vi "Process Motor Status.vi"(8 "error in (no error)":errorcluster, 11 "Motor Error Status":T1) -> (0 "error out":errorcluster, 3 "Error description":string)   [LabVIEW 2012, in "Roboteq.lvlib"]
doc: "Processes the motor status error and outputs a string describing the errors if any."
uses:
  Roboteq.lvlib
  <instrlib>/Dynamixel Motor/Public/Motor Operation/Low Level/Alarm Setting.ctl
  <instrlib>/Dynamixel Motor/Dynamixel Motor.lvlib
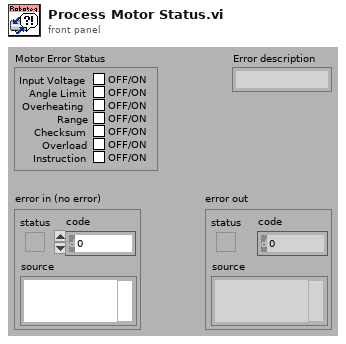
[diagram p1: front panel]
types:
  T1 = typedef "Dynamixel Motor.lvlib/Alarm Setting.ctl" = cluster{"Input Voltage":bool, "Angle Limit":bool, "Overheating ":bool, "Range":bool, "Checksum":bool, "Overload":bool, "Instruction":bool}
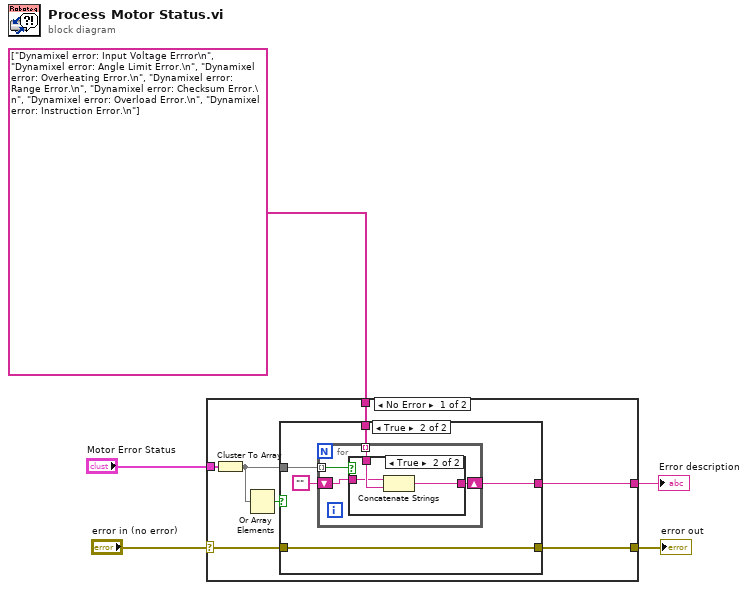
[diagram p0: block diagram]
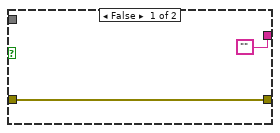
[diagram p2: hidden frame]
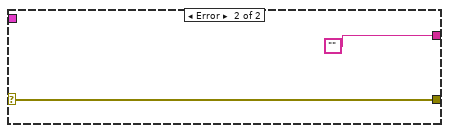
[diagram p4: hidden frame]
diagram:
  n1 = case shown="No Error" "error in (no error)" {
    selector: "error in (no error)" -> [w10 w29]
    tunnel: [w9 w29] -> w4
    tunnel: "Motor Error Status" -> [w12 _]
    tunnel: string[] ["Dynamixel error: Input Voltage Errror\n", "Dynamixel error: Angle Limit Error.\n", "Dynamixel error: Overheating Error.\n", "Dynamixel error: Range Error.\n", "Dynamixel error: Checksum Error.\n", "Dynamixel error: Overload Error.\n", "Dynamixel error: Instruction Error.\n"] -> [w11 _]
    tunnel: [w6 ""] -> w1
    frame No Error {
      n2 = Cluster To Array(cluster=w12) -> (array=w7:bool[])
      n3 = Or Array Elements(Boolean array=w7) -> (logical OR=w8:bool)
      n4 = case shown="True" w8 {
        tunnel: w11 -> [_ w19]
        tunnel: w10 -> [w14 w16]
        tunnel: [w14 w16] -> w9
        tunnel: w7 -> [_ w18]
        tunnel: ["" w15] -> w6
        frame False {
        }
        frame True {
          n5 = for {
            tunnel: w19 -> [w23] mode=indexing
            tunnel: w18 -> [w20] mode=indexing
            shift-right: [w21] -> w15
            shift-left: "" -> [w22]
            n6 = case shown="True" w20 {
              tunnel: w23 -> [_ w27]
              tunnel: w22 -> [w24 w26]
              tunnel: [w24 w25] -> w21
              frame False {
              }
              frame True {
                n7 = Concatenate Strings(w26, w27) -> (w25:string)
              }
            }
          }
        }
      }
    }
    frame Error {
    }
  }
  "error out" <- w4
  "Error description" <- w1
